vi "Sub Super Test.vi"() -> ()   [LabVIEW 2011]
panel:
  in  "Saved Folder:":path=path "D:/userdata/Desktop"
  in  "Stop Control":bool
  in  "Compliance Cluster":T1={"Var1 sweep settings"={"sweep spacing (linear: 0)"=0, "sweep mode"=FALSE, "compliance (V)"=100.0, "compliance (A)"=0.001}, "Var1 sweep settings 2"={"sweep spacing (linear: 0)"=0, "sweep mode"=FALSE, "compliance (V)"=100.0, "compliance (A)"=0.001}, "Var2 step settings 2"={"compliance (A)"=0.001, "compliance (V)"=100.0}, "Var2 step settings"={"compliance (A)"=0.001, "compliance (V)"=100.0}} {"Var2 step settings"."compliance (V)" format="%.2f"; "Var2 step settings"."compliance (A)" format="%^.2e"; "Var2 step settings 2"."compliance (V)" format="%.2f"; "Var2 step settings 2"."compliance (A)" format="%^.2e"; "Var1 sweep settings 2"."compliance (A)" format="%^.2e"; "Var1 sweep settings 2"."compliance (V)" format="%.2f"; "Var1 sweep settings 2"."sweep spacing (linear: 0)" items=["linear", "log 10", "log 25", "log 50"]; "Var1 sweep settings"."compliance (A)" format="%^.2e"; "Var1 sweep settings"."compliance (V)" format="%.2f"; "Var1 sweep settings"."sweep spacing (linear: 0)" items=["linear", "log 10", "log 25", "log 50"]}
  out "Graph Cluster":T2
  in  "TSP Path":path
  in  "TRF Path":path
  out "error out":errorcluster
  out "error in":errorcluster
  out "Wait Cluster":T3 {"Wait Time (s)" format="%.1g"; "Wait Countdown" format="%<%H:%M:%S%1u>t"}
  out "Char Cluster":T4
  in  "TSP Cluster":T5={"Transport"=FALSE, "Start 2"=0.0, "Stop 3"=-60.0, "Step 2"=-1.0, "Start"=0.0, "Step"=-10.0, "Total Points"=7, "Integration Time"=0} {"Integration Time" scale=0.0..2.0; "Step" format="%.2f"; "Start" format="%.2f"; "Step 2" format="%.2f"; "Stop 3" format="%.2f"; "Start 2" format="%.2f"}
  in  "TRF Cluster":T6={"Step 4"=-38.0, "# of Loops"=1.0, "Transfer 2"=TRUE, "Start 4"=-2.0, "Total Points 2"=2, "Start 3"=40.0, "Stop 2"=-40.0, "Step 3"=-1.0, "Loop Step"=0.0, "Integration Time 3"=0, "Loop Wait"=0.0, "First Step"=0.0} {"Loop Wait" format="%<%H:%M:%S>t"; "Integration Time 3" scale=0.0..2.0; "Step 3" format="%.2f"; "Stop 2" format="%.2f"; "Start 3" format="%.2f"; "Start 4" format="%.2f"; "Step 4" format="%.2f"}
  in  "Sample Properties:":T7={"Date Created"=timestamp(3422535498.9557233 s since 1904-01-01), "Material"="Test", "Solvent"="Test", "Concentration"="1", "Method"="Test", "Dielectric (d)"="1", "Index (#)"="1", "Index (ABC)"="A", "Length"="1", "Width"="1", "Surface Treatment"="Test", "Comments"="Test", "T (K)"=0.0} {"Date Created" format="%<%Y/%m/%d>T"}
  out "Status Light":bool
  out "VISA Out":refnum<visa-resource-name>
  in  "VISA In":refnum<visa-resource-name>="GPIB0::17::INSTR"
  # "Vg Step"
  # "Vd Step"
  # "Integration Time"
  # "Sample Properties:"
  # "%"
  # "nm"
  # "Device Properties:"
  # "um"
  # "um"
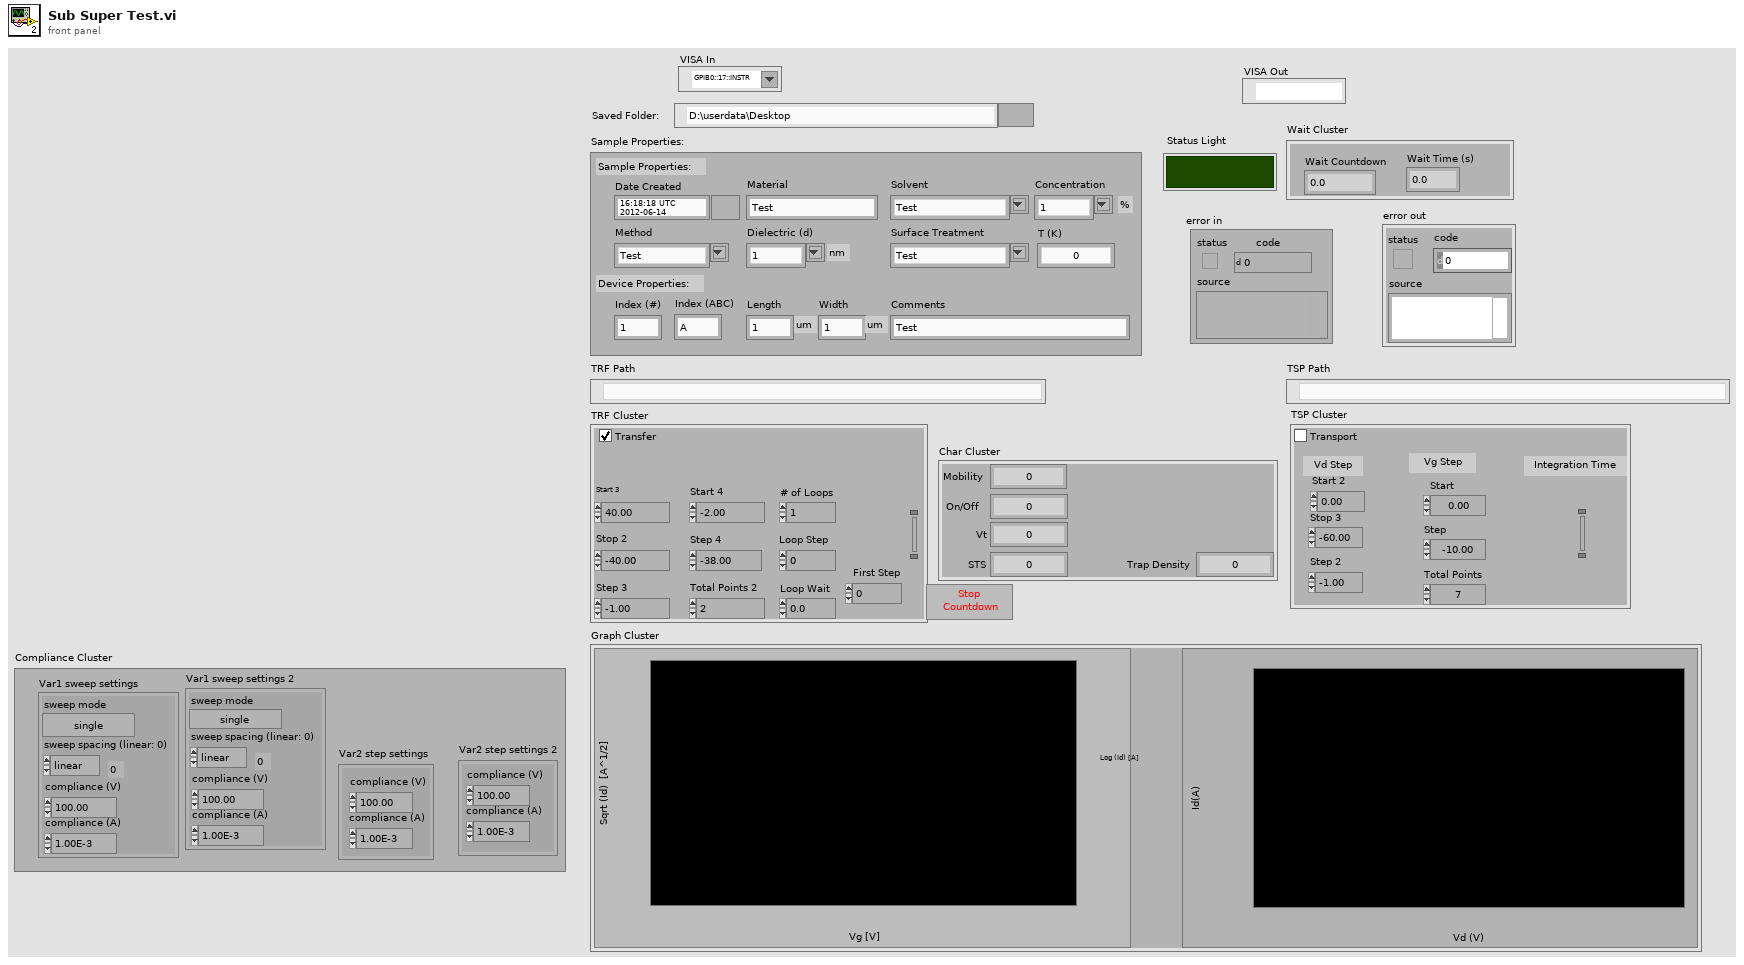
[diagram p1: front panel]
types:
  T1 = cluster{"Var1 sweep settings":cluster{"sweep spacing (linear: 0)":u16, "sweep mode":bool, "compliance (V)":dbl, "compliance (A)":dbl}, "Var1 sweep settings 2":cluster{"sweep spacing (linear: 0)":u16, "sweep mode":bool, "compliance (V)":dbl, "compliance (A)":dbl}, "Var2 step settings 2":cluster{"compliance (A)":dbl, "compliance (V)":dbl}, "Var2 step settings":cluster{"compliance (A)":dbl, "compliance (V)":dbl}}
  T2 = cluster{"Transfer":cluster{dbl[], "trace":dbl[]}[], "Transport":cluster{"trace":dbl[], "trace":dbl[]}}
  T3 = cluster{"Wait Countdown":dbl, "Wait Time (s)":dbl}
  T4 = cluster{"Mobility":dbl, "On/Off ":dbl, "Vt":dbl, "STS":dbl, "Trap Density":dbl}
  T5 = cluster{"Transport":bool, "Start 2":dbl, "Stop 3":dbl, "Step 2":dbl, "Start":dbl, "Step":dbl, "Total Points":u16, "Integration Time":u32}
  T6 = cluster{"Step 4":dbl, "# of Loops":dbl, "Transfer 2":bool, "Start 4":dbl, "Total Points 2":u16, "Start 3":dbl, "Stop 2":dbl, "Step 3":dbl, "Loop Step":dbl, "Integration Time 3":u32, "Loop Wait":dbl, "First Step":dbl}
  T7 = cluster{"Date Created":timestamp, "Material":string, "Solvent":string, "Concentration":string, "Method":string, "Dielectric (d)":string, "Index (#)":string, "Index (ABC)":string, "Length":string, "Width":string, "Surface Treatment":string, "Comments":string, "T (K)":dbl}
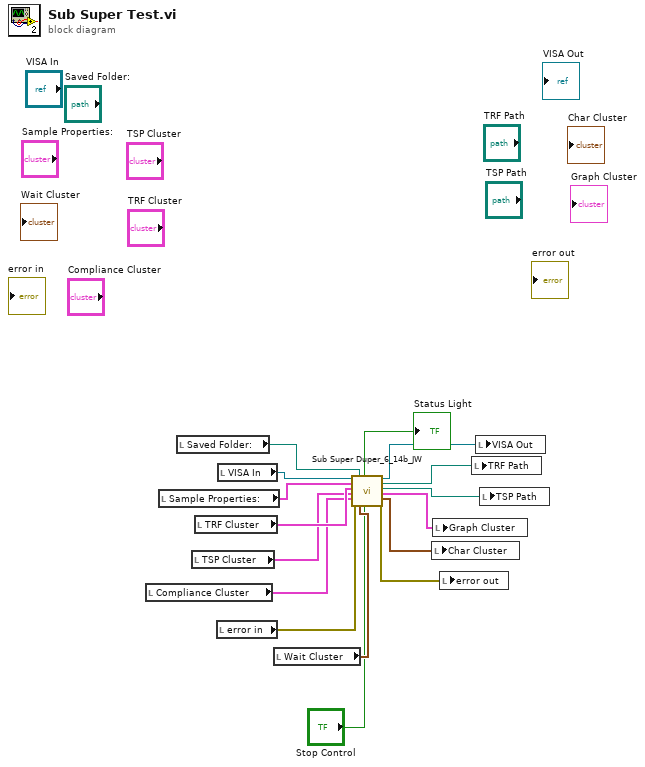
[diagram p0: block diagram]
diagram:
  n1 = local read "Compliance Cluster"() -> (w12:T1)
  n2 = local read "Sample Properties:"() -> (w15:T7)
  n3 = local read "Saved Folder:"() -> (w4:path)
  n4 = local read "TSP Cluster"() -> (w13:T5)
  n5 = local read "TRF Cluster"() -> (w14:T6)
  n6 = local read "error in"() -> (w11:errorcluster)
  n7 = local read "VISA In"() -> (w16:refnum<visa-resource-name>)
  n8 = local read "Wait Cluster"() -> (w10:T3)
  n9 = call "Sub Super Duper_6_14b_JW.vi"("VISA resource name"=w16, "Sample Properties:"=w15, "TRF Cluster"=w14, "TSP Cluster"=w13, "Compliance Cluster"=w12, "error in"=w11, "Saved Folder:"=w4, "Wait Cluster"=w10, "Stop \nCountdown"="Stop Control") -> ("Status Indicator"=→"Status Light":bool, "VISA resource name out"=w9:refnum<visa-resource-name>, "TRF Path"=w2:path, "TSP Path"=w1:path, "Graph Cluster"=w8:T2, "Char Cluster"=w7:T4, "error out"=w6:errorcluster)  [unwired: 4 in]
  n10 = local write "Char Cluster"(w7) -> ()
  n11 = local write "Graph Cluster"(w8) -> ()
  n12 = local write "error out"(w6) -> ()
  n13 = local write "TRF Path"(w2) -> ()
  n14 = local write "VISA Out"(w9) -> ()
  n15 = local write "TSP Path"(w1) -> ()
